vi "DAQ 디지털 버튼, 아날로그 입력 실습(강진성).vi"() -> ()   [LabVIEW 2020]
uses:
  <vilib>/DAQmx/read.llb/DAQmx Read (Analog 2D DBL NChan NSamp).vi
  <vilib>/DAQmx/read.llb/DAQmx Read (Digital 1D Bool 1Chan 1Samp).vi
  <vilib>/DAQmx/create/channels.llb/DAQmx Create Channel (DI-Digital Input).vi
  <vilib>/DAQmx/create/channels.llb/DAQmx Create Channel (AI-Voltage-Basic).vi
  <vilib>/DAQmx/configure/timing.llb/DAQmx Timing (Sample Clock).vi
  <vilib>/DAQmx/miscellaneous.llb/DAQmx Fill In Error Info.vi
panel:
  out "스위치":bool[](array[boolean])
  in  "정지":bool
  out "TMP":dbl[](graph)
  out "PTM":dbl[](graph)
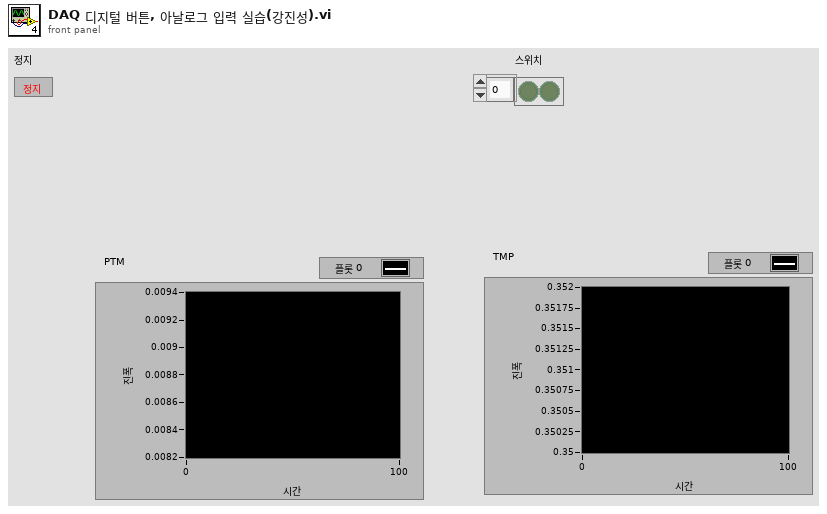
[diagram p1: front panel]
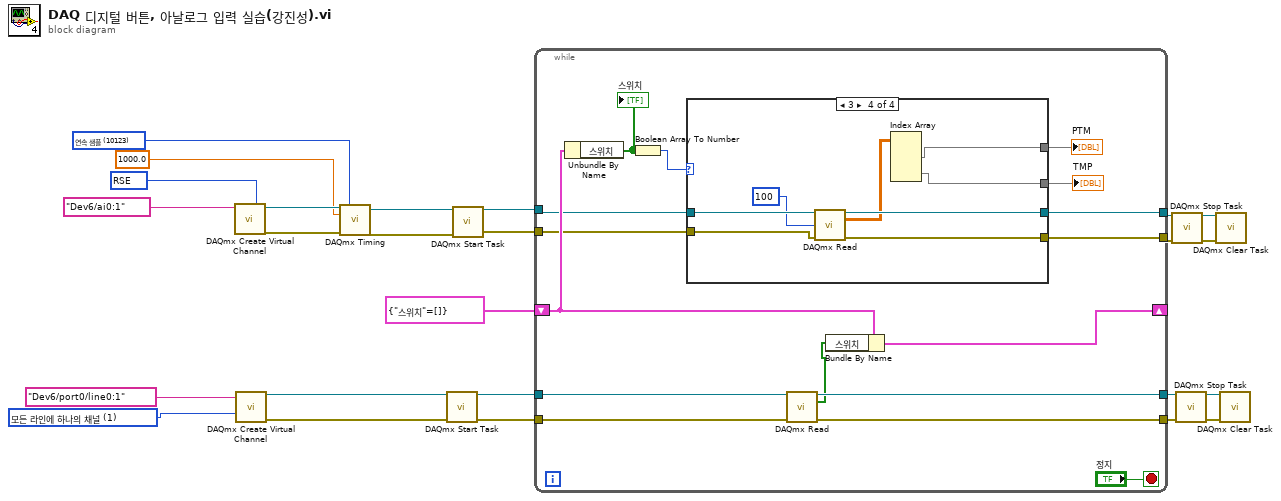
[diagram p0: block diagram]
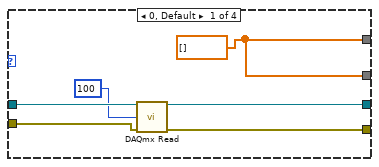
[diagram p2: hidden frame]
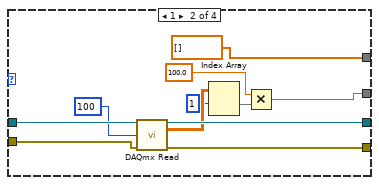
[diagram p3: hidden frame]
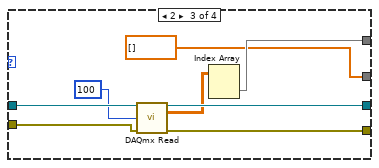
[diagram p4: hidden frame]
diagram:
  w7 = 10123 items=["유한 샘플"=10178, "연속 샘플"=10123, "하드웨어 타이밍에 의한 단일 포인트"=12522] ("sample mode")
  w8 = 10083 items=["기본"=-1, "RSE"=10083, "NRSE"=10078, "차동"=10106, "유사 차동"=12529] ("input terminal configuration")
  w18 = 1 items=["각 라인에 하나의 채널", "모든 라인에 하나의 채널"] ("line grouping")
  n1 = call-poly <vilib>:"DAQmx Create Virtual Channel.vi"("input terminal configuration"=w8, "physical channels"=tag "Dev6/ai0:1") -> ("task out"=w25:refnum<k21>, "error out"=w24:errorcluster)  [unwired: 12 in]
  n2 = call-poly <vilib>:"DAQmx Create Virtual Channel.vi"("lines"=tag "Dev6/port0/line0:1", "line grouping"=w18) -> ("task out"=w17:refnum<k21>, "error out"=w16:errorcluster)  [unwired: 12 in]
  n3 = call-poly <vilib>:"DAQmx Timing.vi"("task/channels in"=w25, "sample mode"=w7, "rate"=1000.0, "error in"=w24) -> ("task out"=w11:refnum<k21>, "error out"=w10:errorcluster)  [unwired: 10 in]
  n4 = call <vilib>:"DAQmx Start Task.vi"("task/channels in"=w17, "error in"=w16) -> ("task out"=w15:refnum<k21>, "error out"=w14:errorcluster)  [unwired: 12 in]
  n5 = call <vilib>:"DAQmx Start Task.vi"("task/channels in"=w11, "error in"=w10) -> ("task out"=w5:refnum<k21>, "error out"=w4:errorcluster)  [unwired: 12 in]
  n6 = while {
    tunnel: w15 -> [w41]
    tunnel: w14 -> [w40]
    tunnel: [w39] -> w13
    tunnel: [w38] -> w12
    tunnel: w5 -> [w32]
    tunnel: w4 -> [w31]
    shift-right: [w37] -> _
    shift-left: cluster{"스위치":bool[]} {"스위치"=[]} -> [w35]
    tunnel: [w30] -> w2
    tunnel: [w29] -> w1
    stop <- "정지" stop-if-true
    n7 = Unbundle By Name(w35) -> ("스위치"=w34:bool[])
    "스위치" <- w34
    n8 = Boolean Array To Number(Boolean array=w34) -> (number=w33:u32)
    n9 = case shown="3" w33 {
      tunnel: w32 -> [w47 w58 w66 w74]
      tunnel: w31 -> [w46 w57 w65 w73]
      tunnel: [w45 w56 w64 w72] -> w30
      tunnel: [w44 w55 w63 w71] -> w29
      tunnel: [w42 w50 dbl[] [] ("data") w67] -> w28
      tunnel: [w42 dbl[] [] ("data") w60 w68] -> w27
      frame 0, Default {
        w42 = dbl[] [] ("data")
        n10 = call-poly <vilib>:"DAQmx Read.vi"("task/channels in"=w47, "number of samples per channel"=100, "error in"=w46) -> ("task out"=w45:refnum<k21>, "error out"=w44:errorcluster)  [unwired: 10 in, 1 out]
      }
      frame 1 {
        n11 = call-poly <vilib>:"DAQmx Read.vi"("task/channels in"=w58, "number of samples per channel"=100, "error in"=w57) -> ("task out"=w56:refnum<k21>, "data"=w53:dbl[][], "error out"=w55:errorcluster)  [unwired: 10 in]
        n12 = Index Array(array=w53, index (row)=1 ("인덱스 (행)")) -> (element=w48:dbl[])  [unwired: 1 in]
        n13 = Multiply(x=100.0, y=w48) -> (x*y=w50:dbl[])
      }
      frame 2 {
        n14 = call-poly <vilib>:"DAQmx Read.vi"("task/channels in"=w66, "number of samples per channel"=100, "error in"=w65) -> ("task out"=w64:refnum<k21>, "data"=w61:dbl[][], "error out"=w63:errorcluster)  [unwired: 10 in]
        n15 = Index Array(array=w61) -> (element=w60:dbl[])  [unwired: 2 in]
      }
      frame 3 {
        n16 = call-poly <vilib>:"DAQmx Read.vi"("task/channels in"=w74, "number of samples per channel"=100, "error in"=w73) -> ("task out"=w72:refnum<k21>, "data"=w69:dbl[][], "error out"=w71:errorcluster)  [unwired: 10 in]
        n17 = Index Array(array=w69) -> (element #1=w68:dbl[], element #2=w67:dbl[])  [unwired: 4 in]
      }
    }
    "PTM" <- w27
    "TMP" <- w28
    n18 = call-poly <vilib>:"DAQmx Read.vi"("task/channels in"=w41, "error in"=w40) -> ("task out"=w39:refnum<k21>, "data"=w36:bool[], "error out"=w38:errorcluster)  [unwired: 11 in]
    n19 = Bundle By Name(cluster=w35, "스위치"=w36) -> (w37:cluster{"스위치":bool[]})
  }
  n20 = call <vilib>:"DAQmx Stop Task.vi"("task/channels in"=w2, "error in"=w1) -> ("task out"=w23:refnum<k21>, "error out"=w22:errorcluster)  [unwired: 12 in]
  n21 = call <vilib>:"DAQmx Stop Task.vi"("task/channels in"=w13, "error in"=w12) -> ("task out"=w21:refnum<k21>, "error out"=w20:errorcluster)  [unwired: 12 in]
  n22 = call <vilib>:"DAQmx Clear Task.vi"("task in"=w23, "error in"=w22) -> ()  [unwired: 13 in, 1 out]
  n23 = call <vilib>:"DAQmx Clear Task.vi"("task in"=w21, "error in"=w20) -> ()  [unwired: 13 in, 1 out]
